vi "AM.vi"(5 "Frequency units":u32(ring) items=["Hz"=1, "KHz"=1000, "MHz"=1000000], 6 "Modulating Depth (%)":dbl(knob) min=0.0 max=120.0 step=1.0 scale=0.0..120.0, 7 "Modulating Frequency":dbl(knob) min=0.0 max=1000.0 step=1.0 scale=2.0..1000.0, 8 "error in":errorcluster, 9 "Signal source":bool, 10 "Waveform":u16(ring) items=["SIN", "SQU", "TRI", "RAMP", "USER"], 11 "Address":string) -> (0 "error out":errorcluster, 2 "Send command":string, 3 "Address (out)":string)   [LabVIEW 2025]
panel:
  # "External"
  # "Both"
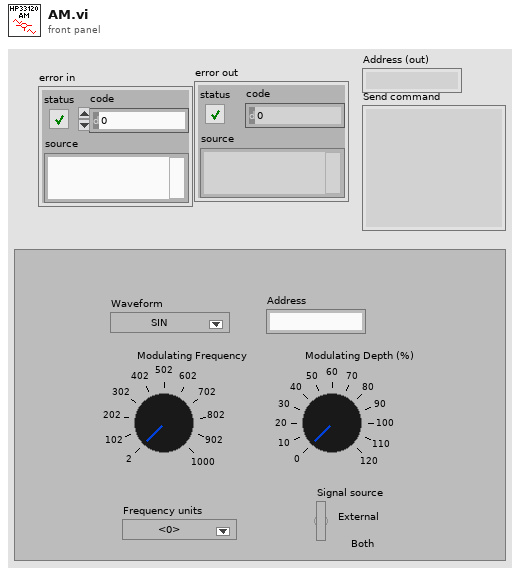
[diagram p1: front panel]
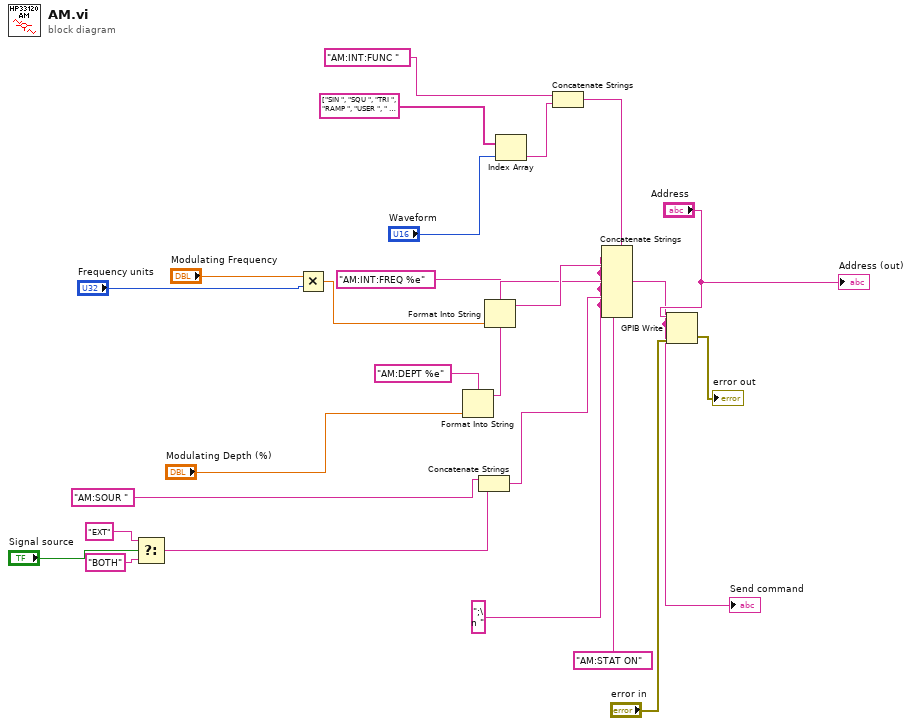
[diagram p0: block diagram]
diagram:
  w10 = ";\n "
  n1 = Select(t="EXT", s="Signal source", f="BOTH") -> (s? t:f=w5:string)
  n2 = Multiply(x="Modulating Frequency", y="Frequency units") -> (x*y=w17:dbl)
  n3 = Format Into String(format string="AM:DEPT %e", "Modulating Depth (%)") -> (resulting string=w12:string)  [unwired: 2 in, 1 out]
  n4 = Concatenate Strings("AM:SOUR ", w5) -> (w11:string)
  n5 = Format Into String(format string="AM:INT:FREQ %e", w17) -> (resulting string=w18:string)  [unwired: 2 in, 1 out]
  n6 = Index Array(array=string[] ["SIN ", "SQU ", "TRI ", "RAMP ", "USER ", " ", "USER "], index="Waveform") -> (element=w15:string)
  n7 = Concatenate Strings("AM:INT:FUNC ", w15) -> (w14:string)
  n8 = Concatenate Strings(w14, w10, w18, w10, w12, w10, w11, w10, "AM:STAT ON") -> (w22:string)
  "Send command" <- w22
  n9 = GPIB Write(0:"Address", 1:w22, 3:"error in") -> (6:→"error out":errorcluster)  [unwired: 2 in, 1 out]
  "Address (out)" <- "Address"
